vi "DSP模拟量输入.vi"() -> ()   [LabVIEW 2010]
panel:
  out "DSP_R_16_5":sgl format="%.2f"
  out "DSP_R_16_4":sgl format="%.2f"
  out "DSP_R_16_3":sgl format="%.2f"
  out "DSP_R_16_2":sgl format="%.2f"
  out "DSP_R_16_1":sgl format="%.2f"
  out "DSP_R_15_5":sgl format="%.2f"
  out "DSP_R_15_4":sgl format="%.2f"
  out "DSP_R_15_3":sgl format="%.2f"
  out "DSP_R_15_2":sgl format="%.2f"
  out "DSP_R_15_1":sgl format="%.2f"
  out "DSP_R_14_5":sgl format="%.2f"
  out "DSP_R_14_4":sgl format="%.2f"
  out "DSP_R_14_3":sgl format="%.2f"
  out "DSP_R_14_2":sgl format="%.2f"
  out "DSP_R_14_1":sgl format="%.2f"
  out "DSP_R_13_5":sgl format="%.2f"
  out "DSP_R_13_4":sgl format="%.2f"
  out "DSP_R_13_3":sgl format="%.2f"
  out "DSP_R_13_2":sgl format="%.2f"
  out "DSP_R_13_1":sgl format="%.2f"
  out "DSP_R_12_5":sgl format="%.2f"
  out "DSP_R_12_4":sgl format="%.2f"
  out "DSP_R_12_3":sgl format="%.2f"
  out "DSP_R_12_2":sgl format="%.2f"
  out "DSP_R_12_1":sgl format="%.2f"
  out "DSP_R_11_5":sgl format="%.2f"
  out "DSP_R_11_4":sgl format="%.2f"
  out "DSP_R_11_3":sgl format="%.2f"
  out "DSP_R_11_2":sgl format="%.2f"
  out "DSP_R_11_1":sgl format="%.2f"
  out "DSP_R_10_5":sgl format="%.2f"
  out "DSP_R_10_4":sgl format="%.2f"
  out "DSP_R_10_3":sgl format="%.2f"
  out "DSP_R_10_2":sgl format="%.2f"
  out "DSP_R_10_1":sgl format="%.2f"
  out "DSP_R_9_5":sgl format="%.2f"
  out "DSP_R_9_4":sgl format="%.2f"
  out "DSP_R_9_3":sgl format="%.2f"
  out "DSP_R_9_2":sgl format="%.2f"
  out "DSP_R_9_1":sgl format="%.2f"
  out "DSP_R_8_5":sgl format="%.2f"
  out "DSP_R_8_4":sgl format="%.2f"
  out "DSP_R_8_3":sgl format="%.2f"
  out "DSP_R_8_2":sgl format="%.2f"
  out "DSP_R_8_1":sgl format="%.2f"
  out "DSP_R_7_5":sgl format="%.2f"
  out "DSP_R_7_4":sgl format="%.2f"
  out "DSP_R_7_3":sgl format="%.2f"
  out "DSP_R_7_2":sgl format="%.2f"
  out "DSP_R_7_1":sgl format="%.2f"
  out "DSP_R_6_5":sgl format="%.2f"
  out "DSP_R_6_4":sgl format="%.2f"
  out "DSP_R_6_3":sgl format="%.2f"
  out "DSP_R_6_2":sgl format="%.2f"
  out "DSP_R_6_1":sgl format="%.2f"
  out "DSP_R_5_5":sgl format="%.2f"
  out "DSP_R_5_4":sgl format="%.2f"
  out "DSP_R_5_3":sgl format="%.2f"
  out "DSP_R_5_2":sgl format="%.2f"
  out "DSP_R_5_1":sgl format="%.2f"
  out "DSP_R_4_5":sgl format="%.2f"
  out "DSP_R_4_4":sgl format="%.2f"
  out "DSP_R_4_3":sgl format="%.2f"
  out "DSP_R_4_2":sgl format="%.2f"
  out "DSP_R_4_1":sgl format="%.2f"
  out "DSP_R_3_5":sgl format="%.2f"
  out "DSP_R_3_4":sgl format="%.2f"
  out "DSP_R_3_3":sgl format="%.2f"
  out "DSP_R_3_2":sgl format="%.2f"
  out "DSP_R_3_1":sgl format="%.2f"
  out "DSP_R_2_5":sgl format="%.2f"
  out "DSP_R_2_4":sgl format="%.2f"
  out "DSP_R_2_3":sgl format="%.2f"
  out "DSP_R_2_2":sgl format="%.2f"
  out "DSP_R_2_1":sgl format="%.2f"
  out "DSP_R_1_5":sgl format="%.2f"
  out "DSP_R_1_4":sgl format="%.2f"
  out "DSP_R_1_3":sgl format="%.2f"
  out "DSP_R_1_2":sgl format="%.2f"
  out "DSP_R_1_1":sgl format="%.2f"
  out "合格？":bool[][](array[boolean])
  out "开始时间":dbl format="%#.0f"
  out "测试结论":string
  out "light_16":bool
  out "light_15":bool
  out "light_14":bool
  out "light_13":bool
  out "light_12":bool
  out "light_11":bool
  out "light_10":bool
  out "light_9":bool
  out "light_8":bool
  out "light_7":bool
  out "light_6":bool
  out "light_5":bool
  out "light_4":bool
  out "light_3":bool
  out "light_2":bool
  out "light_1":bool
  out "退出？":bool
  in  "btn_反选":bool
  in  "btn_全选":bool
  in  "DSP_16_5":sgl format="%.2f"
  in  "DSP_16_4":sgl format="%.2f"
  in  "DSP_16_3":sgl format="%.2f"
  in  "DSP_16_2":sgl format="%.2f"
  in  "DSP_16_1":sgl format="%.2f"
  in  "DSP_15_5":sgl format="%.2f"
  in  "DSP_15_4":sgl format="%.2f"
  in  "DSP_15_3":sgl format="%.2f"
  in  "DSP_15_2":sgl format="%.2f"
  in  "单选_DSP_16":bool
  in  "单选_DSP_15":bool
  in  "DSP_15_1":sgl format="%.2f"
  in  "DSP_14_5":sgl format="%.2f"
  in  "DSP_14_4":sgl format="%.2f"
  in  "DSP_14_3":sgl format="%.2f"
  in  "DSP_14_2":sgl format="%.2f"
  in  "DSP_6_14":sgl format="%.2f"
  in  "DSP_13_5":sgl format="%.2f"
  in  "DSP_13_4":sgl format="%.2f"
  in  "DSP_13_3":sgl format="%.2f"
  in  "DSP_13_2":sgl format="%.2f"
  in  "单选_DSP_14":bool
  in  "单选_DSP_13":bool
  in  "DSP_13_1":sgl format="%.2f"
  in  "DSP_12_5":sgl format="%.2f"
  in  "DSP_12_4":sgl format="%.2f"
  in  "DSP_12_3":sgl format="%.2f"
  in  "DSP_12_2":sgl format="%.2f"
  in  "DSP_12_1":sgl format="%.2f"
  in  "DSP_11_5":sgl format="%.2f"
  in  "DSP_11_4":sgl format="%.2f"
  in  "DSP_11_3":sgl format="%.2f"
  in  "DSP_11_2":sgl format="%.2f"
  in  "单选_DSP_12":bool
  in  "单选_DSP_11":bool
  in  "DSP_11_1":sgl format="%.2f"
  in  "DSP_10_5":sgl format="%.2f"
  in  "DSP_10_4":sgl format="%.2f"
  in  "DSP_10_3":sgl format="%.2f"
  in  "DSP_10_2":sgl format="%.2f"
  in  "DSP_10_1":sgl format="%.2f"
  in  "DSP_9_5":sgl format="%.2f"
  in  "DSP_9_4":sgl format="%.2f"
  in  "DSP_9_3":sgl format="%.2f"
  in  "DSP_9_2":sgl format="%.2f"
  in  "单选_DSP_10":bool
  in  "单选_DSP_9":bool
  in  "DSP_9_1":sgl format="%.2f"
  in  "DSP_8_5":sgl format="%.2f"
  in  "DSP_8_4":sgl format="%.2f"
  in  "DSP_8_3":sgl format="%.2f"
  in  "DSP_8_2":sgl format="%.2f"
  in  "DSP_8_1":sgl format="%.2f"
  in  "DSP_7_5":sgl format="%.2f"
  in  "DSP_7_4":sgl format="%.2f"
  in  "DSP_7_3":sgl format="%.2f"
  in  "DSP_7_2":sgl format="%.2f"
  in  "单选_DSP_8":bool
  in  "单选_DSP_7":bool
  in  "DSP_7_1":sgl format="%.2f"
  in  "DSP_6_5":sgl format="%.2f"
  in  "DSP_6_4":sgl format="%.2f"
  in  "DSP_6_3":sgl format="%.2f"
  in  "DSP_6_2":sgl format="%.2f"
  in  "DSP_6_1":sgl format="%.2f"
  in  "DSP_5_5":sgl format="%.2f"
  in  "DSP_5_4":sgl format="%.2f"
  in  "DSP_5_3":sgl format="%.2f"
  in  "DSP_5_2":sgl format="%.2f"
  in  "单选_DSP_6":bool
  in  "单选_DSP_5":bool
  in  "DSP_5_1":sgl format="%.2f"
  in  "DSP_4_5":sgl format="%.2f"
  in  "DSP_4_4":sgl format="%.2f"
  in  "DSP_4_3":sgl format="%.2f"
  in  "DSP_4_2":sgl format="%.2f"
  in  "DSP_4_1":sgl format="%.2f"
  in  "DSP_3_5":sgl format="%.2f"
  in  "DSP_3_4":sgl format="%.2f"
  in  "DSP_3_3":sgl format="%.2f"
  in  "DSP_3_2":sgl format="%.2f"
  in  "单选_DSP_4":bool
  in  "单选_DSP_3":bool
  in  "DSP_3_1":sgl format="%.2f"
  in  "DSP_2_5":sgl format="%.2f"
  in  "DSP_2_4":sgl format="%.2f"
  in  "DSP_2_3":sgl format="%.2f"
  in  "DSP_2_2":sgl format="%.2f"
  in  "DSP_2_1":sgl format="%.2f"
  in  "DSP_1_5":sgl format="%.2f"
  in  "DSP_1_4":sgl format="%.2f"
  in  "DSP_1_3":sgl format="%.2f"
  in  "DSP_1_2":sgl format="%.2f"
  in  "单选_DSP_2":bool
  in  "单选_DSP_1":bool
  in  "DSP_1_1":sgl format="%.2f"
  in  "btn_取消":bool
  in  "btn_开始测试":bool
  # "第1路"
  # "输入值："
  # "输入值："
  # "第2路"
  # "第3路"
  # "输入值："
  # "输入值："
  # "第4路"
  # "第5路"
  # "输入值："
  # "输入值："
  # "第6路"
  # "第7路"
  # "输入值："
  # "输入值："
  # "第8路"
  # "第9路"
  # "输入值："
  # "输入值："
  # "第10路"
  # "第11路"
  # "输入值："
  # "输入值："
  # "第12路"
  # "第13路"
  # "输入值："
  # "输入值："
  # "第14路"
  # "第15路"
  # "输入值："
  # "输入值："
  # "第16路"
  # "测试结论："
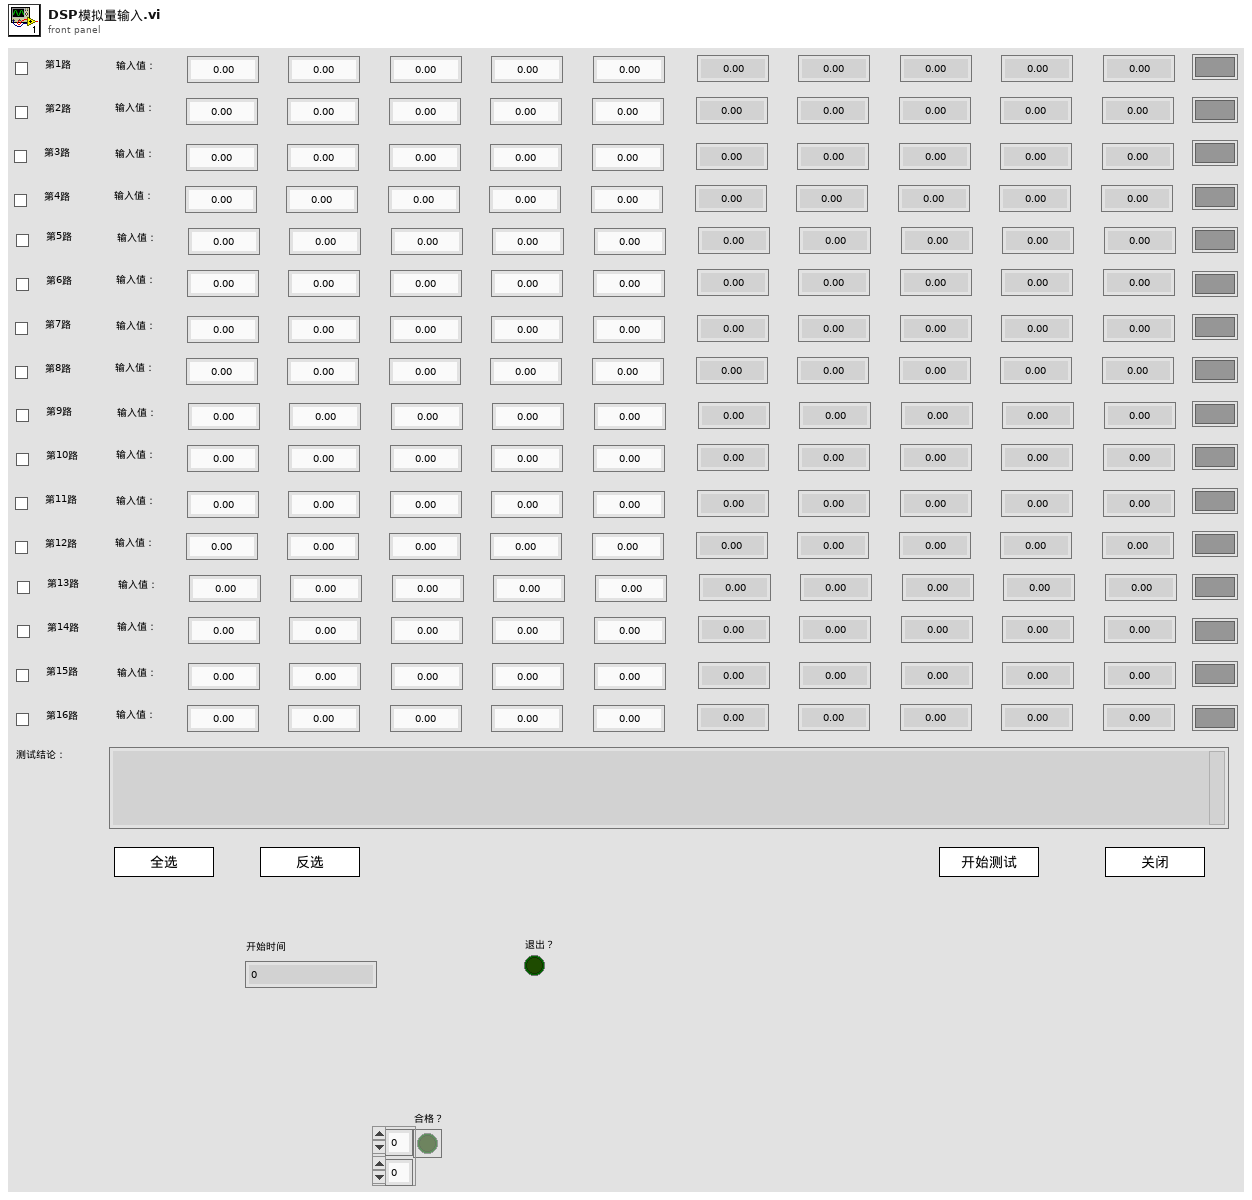
[diagram p1: front panel]
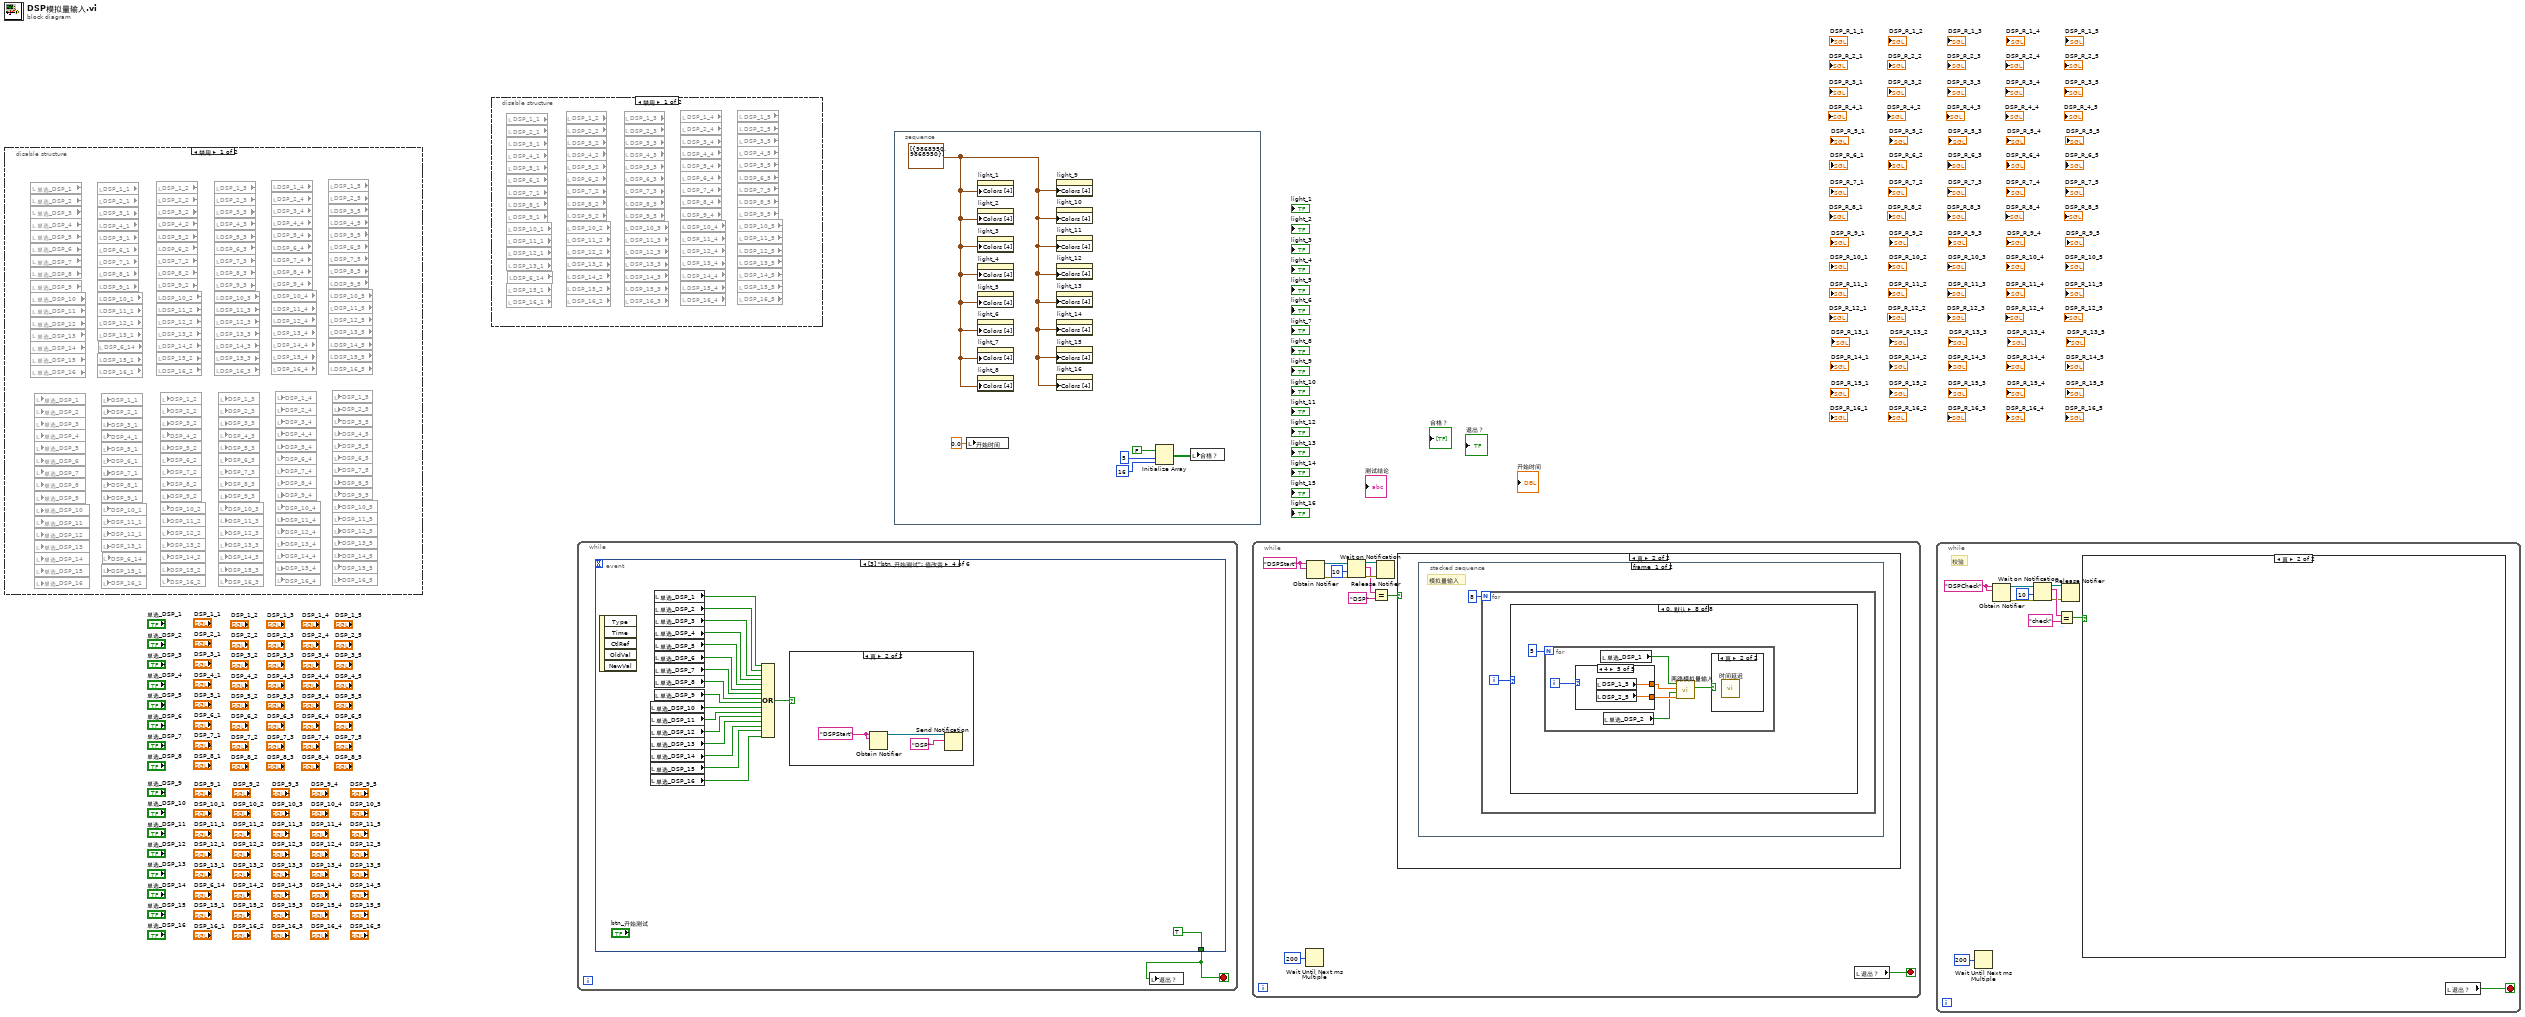
[diagram p0: block diagram]
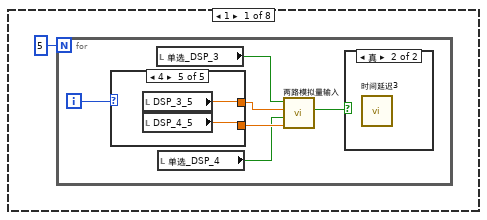
[diagram p5: hidden frame]
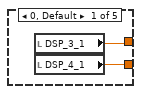
[diagram p7: hidden frame]
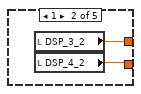
[diagram p8: hidden frame]
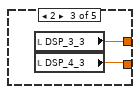
[diagram p9: hidden frame]
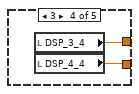
[diagram p10: hidden frame]
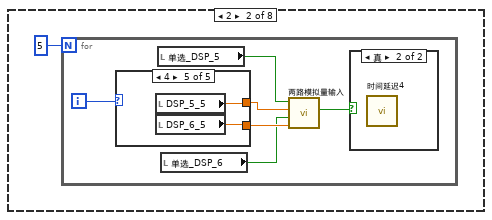
[diagram p11: hidden frame]
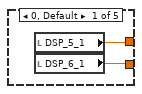
[diagram p13: hidden frame]
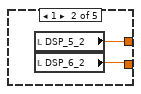
[diagram p14: hidden frame]
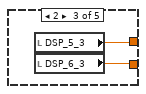
[diagram p15: hidden frame]
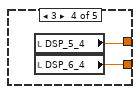
[diagram p16: hidden frame]
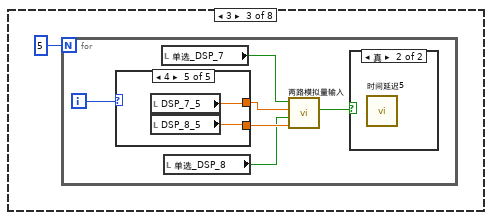
[diagram p17: hidden frame]
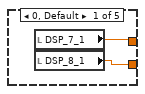
[diagram p19: hidden frame]
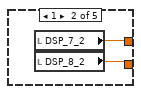
[diagram p20: hidden frame]
diagram:
  n1 = disable-structure shown="禁用" {
    frame Disabled {
      n2 = local read "单选_DSP_1"() -> ()  [unwired: 1 out]
      n3 = local read "单选_DSP_2"() -> ()  [unwired: 1 out]
      n4 = local read "单选_DSP_3"() -> ()  [unwired: 1 out]
      n5 = local read "单选_DSP_4"() -> ()  [unwired: 1 out]
      n6 = local read "单选_DSP_5"() -> ()  [unwired: 1 out]
      n7 = local read "单选_DSP_6"() -> ()  [unwired: 1 out]
      n8 = local read "单选_DSP_7"() -> ()  [unwired: 1 out]
      n9 = local read "单选_DSP_8"() -> ()  [unwired: 1 out]
      n10 = local read "单选_DSP_9"() -> ()  [unwired: 1 out]
      n11 = local read "单选_DSP_10"() -> ()  [unwired: 1 out]
      n12 = local read "单选_DSP_11"() -> ()  [unwired: 1 out]
      n13 = local read "单选_DSP_12"() -> ()  [unwired: 1 out]
      n14 = local read "单选_DSP_13"() -> ()  [unwired: 1 out]
      n15 = local read "单选_DSP_14"() -> ()  [unwired: 1 out]
      n16 = local read "单选_DSP_15"() -> ()  [unwired: 1 out]
      n17 = local read "单选_DSP_16"() -> ()  [unwired: 1 out]
      n18 = local read "单选_DSP_1"() -> ()  [unwired: 1 in]
      n19 = local read "单选_DSP_2"() -> ()  [unwired: 1 in]
      n20 = local read "单选_DSP_3"() -> ()  [unwired: 1 in]
      n21 = local read "单选_DSP_4"() -> ()  [unwired: 1 in]
      n22 = local read "单选_DSP_5"() -> ()  [unwired: 1 in]
      n23 = local read "单选_DSP_6"() -> ()  [unwired: 1 in]
      n24 = local read "单选_DSP_7"() -> ()  [unwired: 1 in]
      n25 = local read "单选_DSP_8"() -> ()  [unwired: 1 in]
      n26 = local read "单选_DSP_9"() -> ()  [unwired: 1 in]
      n27 = local read "单选_DSP_10"() -> ()  [unwired: 1 in]
      n28 = local read "单选_DSP_11"() -> ()  [unwired: 1 in]
      n29 = local read "单选_DSP_12"() -> ()  [unwired: 1 in]
      n30 = local read "单选_DSP_13"() -> ()  [unwired: 1 in]
      n31 = local read "单选_DSP_14"() -> ()  [unwired: 1 in]
      n32 = local read "单选_DSP_15"() -> ()  [unwired: 1 in]
      n33 = local read "单选_DSP_16"() -> ()  [unwired: 1 in]
      n34 = local read "DSP_1_1"() -> ()  [unwired: 1 out]
      n35 = local read "DSP_2_1"() -> ()  [unwired: 1 out]
      n36 = local read "DSP_3_1"() -> ()  [unwired: 1 out]
      n37 = local read "DSP_4_1"() -> ()  [unwired: 1 out]
      n38 = local read "DSP_5_1"() -> ()  [unwired: 1 out]
      n39 = local read "DSP_6_1"() -> ()  [unwired: 1 out]
      n40 = local read "DSP_7_1"() -> ()  [unwired: 1 out]
      n41 = local read "DSP_8_1"() -> ()  [unwired: 1 out]
      n42 = local read "DSP_9_1"() -> ()  [unwired: 1 out]
      n43 = local read "DSP_10_1"() -> ()  [unwired: 1 out]
      n44 = local read "DSP_11_1"() -> ()  [unwired: 1 out]
      n45 = local read "DSP_12_1"() -> ()  [unwired: 1 out]
      n46 = local read "DSP_13_1"() -> ()  [unwired: 1 out]
      n47 = local read "DSP_15_1"() -> ()  [unwired: 1 out]
      n48 = local read "DSP_16_1"() -> ()  [unwired: 1 out]
      n49 = local read "DSP_6_14"() -> ()  [unwired: 1 out]
      n50 = local read "DSP_1_1"() -> ()  [unwired: 1 in]
      n51 = local read "DSP_2_1"() -> ()  [unwired: 1 in]
      n52 = local read "DSP_3_1"() -> ()  [unwired: 1 in]
      n53 = local read "DSP_4_1"() -> ()  [unwired: 1 in]
      n54 = local read "DSP_5_1"() -> ()  [unwired: 1 in]
      n55 = local read "DSP_6_1"() -> ()  [unwired: 1 in]
      n56 = local read "DSP_7_1"() -> ()  [unwired: 1 in]
      n57 = local read "DSP_8_1"() -> ()  [unwired: 1 in]
      n58 = local read "DSP_9_1"() -> ()  [unwired: 1 in]
      n59 = local read "DSP_10_1"() -> ()  [unwired: 1 in]
      n60 = local read "DSP_11_1"() -> ()  [unwired: 1 in]
      n61 = local read "DSP_12_1"() -> ()  [unwired: 1 in]
      n62 = local read "DSP_13_1"() -> ()  [unwired: 1 in]
      n63 = local read "DSP_15_1"() -> ()  [unwired: 1 in]
      n64 = local read "DSP_16_1"() -> ()  [unwired: 1 in]
      n65 = local read "DSP_6_14"() -> ()  [unwired: 1 in]
      n66 = local read "DSP_1_2"() -> ()  [unwired: 1 out]
      n67 = local read "DSP_2_2"() -> ()  [unwired: 1 out]
      n68 = local read "DSP_3_2"() -> ()  [unwired: 1 out]
      n69 = local read "DSP_4_2"() -> ()  [unwired: 1 out]
      n70 = local read "DSP_5_2"() -> ()  [unwired: 1 out]
      n71 = local read "DSP_6_2"() -> ()  [unwired: 1 out]
      n72 = local read "DSP_7_2"() -> ()  [unwired: 1 out]
      n73 = local read "DSP_8_2"() -> ()  [unwired: 1 out]
      n74 = local read "DSP_9_2"() -> ()  [unwired: 1 out]
      n75 = local read "DSP_10_2"() -> ()  [unwired: 1 out]
      n76 = local read "DSP_11_2"() -> ()  [unwired: 1 out]
      n77 = local read "DSP_12_2"() -> ()  [unwired: 1 out]
      n78 = local read "DSP_13_2"() -> ()  [unwired: 1 out]
      n79 = local read "DSP_14_2"() -> ()  [unwired: 1 out]
      n80 = local read "DSP_15_2"() -> ()  [unwired: 1 out]
      n81 = local read "DSP_16_2"() -> ()  [unwired: 1 out]
      n82 = local read "DSP_1_2"() -> ()  [unwired: 1 in]
      n83 = local read "DSP_2_2"() -> ()  [unwired: 1 in]
      n84 = local read "DSP_3_2"() -> ()  [unwired: 1 in]
      n85 = local read "DSP_4_2"() -> ()  [unwired: 1 in]
      n86 = local read "DSP_5_2"() -> ()  [unwired: 1 in]
      n87 = local read "DSP_6_2"() -> ()  [unwired: 1 in]
      n88 = local read "DSP_7_2"() -> ()  [unwired: 1 in]
      n89 = local read "DSP_8_2"() -> ()  [unwired: 1 in]
      n90 = local read "DSP_9_2"() -> ()  [unwired: 1 in]
      n91 = local read "DSP_10_2"() -> ()  [unwired: 1 in]
      n92 = local read "DSP_11_2"() -> ()  [unwired: 1 in]
      n93 = local read "DSP_12_2"() -> ()  [unwired: 1 in]
      n94 = local read "DSP_13_2"() -> ()  [unwired: 1 in]
      n95 = local read "DSP_14_2"() -> ()  [unwired: 1 in]
      n96 = local read "DSP_15_2"() -> ()  [unwired: 1 in]
      n97 = local read "DSP_16_2"() -> ()  [unwired: 1 in]
      n98 = local read "DSP_1_3"() -> ()  [unwired: 1 out]
      n99 = local read "DSP_2_3"() -> ()  [unwired: 1 out]
      n100 = local read "DSP_3_3"() -> ()  [unwired: 1 out]
      n101 = local read "DSP_4_3"() -> ()  [unwired: 1 out]
      n102 = local read "DSP_5_3"() -> ()  [unwired: 1 out]
      n103 = local read "DSP_6_3"() -> ()  [unwired: 1 out]
      n104 = local read "DSP_7_3"() -> ()  [unwired: 1 out]
      n105 = local read "DSP_8_3"() -> ()  [unwired: 1 out]
      n106 = local read "DSP_9_3"() -> ()  [unwired: 1 out]
      n107 = local read "DSP_10_3"() -> ()  [unwired: 1 out]
      n108 = local read "DSP_11_3"() -> ()  [unwired: 1 out]
      n109 = local read "DSP_12_3"() -> ()  [unwired: 1 out]
      n110 = local read "DSP_13_3"() -> ()  [unwired: 1 out]
      n111 = local read "DSP_14_3"() -> ()  [unwired: 1 out]
      n112 = local read "DSP_15_3"() -> ()  [unwired: 1 out]
      n113 = local read "DSP_16_3"() -> ()  [unwired: 1 out]
      n114 = local read "DSP_1_3"() -> ()  [unwired: 1 in]
      n115 = local read "DSP_2_3"() -> ()  [unwired: 1 in]
      n116 = local read "DSP_3_3"() -> ()  [unwired: 1 in]
      n117 = local read "DSP_4_3"() -> ()  [unwired: 1 in]
      n118 = local read "DSP_5_3"() -> ()  [unwired: 1 in]
      n119 = local read "DSP_6_3"() -> ()  [unwired: 1 in]
      n120 = local read "DSP_7_3"() -> ()  [unwired: 1 in]
      n121 = local read "DSP_8_3"() -> ()  [unwired: 1 in]
      n122 = local read "DSP_9_3"() -> ()  [unwired: 1 in]
      n123 = local read "DSP_10_3"() -> ()  [unwired: 1 in]
      n124 = local read "DSP_11_3"() -> ()  [unwired: 1 in]
      n125 = local read "DSP_12_3"() -> ()  [unwired: 1 in]
      n126 = local read "DSP_13_3"() -> ()  [unwired: 1 in]
      n127 = local read "DSP_14_3"() -> ()  [unwired: 1 in]
      n128 = local read "DSP_15_3"() -> ()  [unwired: 1 in]
      n129 = local read "DSP_16_3"() -> ()  [unwired: 1 in]
      n130 = local read "DSP_1_4"() -> ()  [unwired: 1 out]
      n131 = local read "DSP_2_4"() -> ()  [unwired: 1 out]
      n132 = local read "DSP_3_4"() -> ()  [unwired: 1 out]
      n133 = local read "DSP_4_4"() -> ()  [unwired: 1 out]
      n134 = local read "DSP_5_4"() -> ()  [unwired: 1 out]
      n135 = local read "DSP_6_4"() -> ()  [unwired: 1 out]
      n136 = local read "DSP_7_4"() -> ()  [unwired: 1 out]
      n137 = local read "DSP_8_4"() -> ()  [unwired: 1 out]
      n138 = local read "DSP_9_4"() -> ()  [unwired: 1 out]
      n139 = local read "DSP_10_4"() -> ()  [unwired: 1 out]
      n140 = local read "DSP_11_4"() -> ()  [unwired: 1 out]
      n141 = local read "DSP_12_4"() -> ()  [unwired: 1 out]
      n142 = local read "DSP_13_4"() -> ()  [unwired: 1 out]
      n143 = local read "DSP_14_4"() -> ()  [unwired: 1 out]
      n144 = local read "DSP_15_4"() -> ()  [unwired: 1 out]
      n145 = local read "DSP_16_4"() -> ()  [unwired: 1 out]
      n146 = local read "DSP_1_4"() -> ()  [unwired: 1 in]
      n147 = local read "DSP_2_4"() -> ()  [unwired: 1 in]
      n148 = local read "DSP_3_4"() -> ()  [unwired: 1 in]
      n149 = local read "DSP_4_4"() -> ()  [unwired: 1 in]
      n150 = local read "DSP_5_4"() -> ()  [unwired: 1 in]
      n151 = local read "DSP_6_4"() -> ()  [unwired: 1 in]
      n152 = local read "DSP_7_4"() -> ()  [unwired: 1 in]
      n153 = local read "DSP_8_4"() -> ()  [unwired: 1 in]
      n154 = local read "DSP_9_4"() -> ()  [unwired: 1 in]
      n155 = local read "DSP_10_4"() -> ()  [unwired: 1 in]
      n156 = local read "DSP_11_4"() -> ()  [unwired: 1 in]
      n157 = local read "DSP_12_4"() -> ()  [unwired: 1 in]
      n158 = local read "DSP_13_4"() -> ()  [unwired: 1 in]
      n159 = local read "DSP_14_4"() -> ()  [unwired: 1 in]
      n160 = local read "DSP_15_4"() -> ()  [unwired: 1 in]
      n161 = local read "DSP_16_4"() -> ()  [unwired: 1 in]
      n162 = local read "DSP_1_5"() -> ()  [unwired: 1 out]
      n163 = local read "DSP_2_5"() -> ()  [unwired: 1 out]
      n164 = local read "DSP_3_5"() -> ()  [unwired: 1 out]
      n165 = local read "DSP_4_5"() -> ()  [unwired: 1 out]
      n166 = local read "DSP_5_5"() -> ()  [unwired: 1 out]
      n167 = local read "DSP_6_5"() -> ()  [unwired: 1 out]
      n168 = local read "DSP_7_5"() -> ()  [unwired: 1 out]
      n169 = local read "DSP_8_5"() -> ()  [unwired: 1 out]
      n170 = local read "DSP_9_5"() -> ()  [unwired: 1 out]
      n171 = local read "DSP_10_5"() -> ()  [unwired: 1 out]
      n172 = local read "DSP_11_5"() -> ()  [unwired: 1 out]
      n173 = local read "DSP_12_5"() -> ()  [unwired: 1 out]
      n174 = local read "DSP_13_5"() -> ()  [unwired: 1 out]
      n175 = local read "DSP_14_5"() -> ()  [unwired: 1 out]
      n176 = local read "DSP_15_5"() -> ()  [unwired: 1 out]
      n177 = local read "DSP_16_5"() -> ()  [unwired: 1 out]
      n178 = local read "DSP_1_5"() -> ()  [unwired: 1 in]
      n179 = local read "DSP_2_5"() -> ()  [unwired: 1 in]
      n180 = local read "DSP_3_5"() -> ()  [unwired: 1 in]
      n181 = local read "DSP_4_5"() -> ()  [unwired: 1 in]
      n182 = local read "DSP_5_5"() -> ()  [unwired: 1 in]
      n183 = local read "DSP_6_5"() -> ()  [unwired: 1 in]
      n184 = local read "DSP_7_5"() -> ()  [unwired: 1 in]
      n185 = local read "DSP_8_5"() -> ()  [unwired: 1 in]
      n186 = local read "DSP_9_5"() -> ()  [unwired: 1 in]
      n187 = local read "DSP_10_5"() -> ()  [unwired: 1 in]
      n188 = local read "DSP_11_5"() -> ()  [unwired: 1 in]
      n189 = local read "DSP_12_5"() -> ()  [unwired: 1 in]
      n190 = local read "DSP_13_5"() -> ()  [unwired: 1 in]
      n191 = local read "DSP_14_5"() -> ()  [unwired: 1 in]
      n192 = local read "DSP_15_5"() -> ()  [unwired: 1 in]
      n193 = local read "DSP_16_5"() -> ()  [unwired: 1 in]
    }
    frame Enabled {
    }
  }
  n194 = disable-structure shown="禁用" {
    frame Disabled {
      n195 = local read "DSP_1_1"() -> ()  [unwired: 1 out]
      n196 = local read "DSP_2_1"() -> ()  [unwired: 1 out]
      n197 = local read "DSP_3_1"() -> ()  [unwired: 1 out]
      n198 = local read "DSP_4_1"() -> ()  [unwired: 1 out]
      n199 = local read "DSP_5_1"() -> ()  [unwired: 1 out]
      n200 = local read "DSP_6_1"() -> ()  [unwired: 1 out]
      n201 = local read "DSP_7_1"() -> ()  [unwired: 1 out]
      n202 = local read "DSP_8_1"() -> ()  [unwired: 1 out]
      n203 = local read "DSP_9_1"() -> ()  [unwired: 1 out]
      n204 = local read "DSP_10_1"() -> ()  [unwired: 1 out]
      n205 = local read "DSP_11_1"() -> ()  [unwired: 1 out]
      n206 = local read "DSP_12_1"() -> ()  [unwired: 1 out]
      n207 = local read "DSP_13_1"() -> ()  [unwired: 1 out]
      n208 = local read "DSP_15_1"() -> ()  [unwired: 1 out]
      n209 = local read "DSP_16_1"() -> ()  [unwired: 1 out]
      n210 = local read "DSP_6_14"() -> ()  [unwired: 1 out]
      n211 = local read "DSP_1_2"() -> ()  [unwired: 1 out]
      n212 = local read "DSP_2_2"() -> ()  [unwired: 1 out]
      n213 = local read "DSP_3_2"() -> ()  [unwired: 1 out]
      n214 = local read "DSP_4_2"() -> ()  [unwired: 1 out]
      n215 = local read "DSP_5_2"() -> ()  [unwired: 1 out]
      n216 = local read "DSP_6_2"() -> ()  [unwired: 1 out]
      n217 = local read "DSP_7_2"() -> ()  [unwired: 1 out]
      n218 = local read "DSP_8_2"() -> ()  [unwired: 1 out]
      n219 = local read "DSP_9_2"() -> ()  [unwired: 1 out]
      n220 = local read "DSP_10_2"() -> ()  [unwired: 1 out]
      n221 = local read "DSP_11_2"() -> ()  [unwired: 1 out]
      n222 = local read "DSP_12_2"() -> ()  [unwired: 1 out]
      n223 = local read "DSP_13_2"() -> ()  [unwired: 1 out]
      n224 = local read "DSP_14_2"() -> ()  [unwired: 1 out]
      n225 = local read "DSP_15_2"() -> ()  [unwired: 1 out]
      n226 = local read "DSP_16_2"() -> ()  [unwired: 1 out]
      n227 = local read "DSP_1_3"() -> ()  [unwired: 1 out]
      n228 = local read "DSP_2_3"() -> ()  [unwired: 1 out]
      n229 = local read "DSP_3_3"() -> ()  [unwired: 1 out]
      n230 = local read "DSP_4_3"() -> ()  [unwired: 1 out]
      n231 = local read "DSP_5_3"() -> ()  [unwired: 1 out]
      n232 = local read "DSP_6_3"() -> ()  [unwired: 1 out]
      n233 = local read "DSP_7_3"() -> ()  [unwired: 1 out]
      n234 = local read "DSP_8_3"() -> ()  [unwired: 1 out]
      n235 = local read "DSP_9_3"() -> ()  [unwired: 1 out]
      n236 = local read "DSP_10_3"() -> ()  [unwired: 1 out]
      n237 = local read "DSP_11_3"() -> ()  [unwired: 1 out]
      n238 = local read "DSP_12_3"() -> ()  [unwired: 1 out]
      n239 = local read "DSP_13_3"() -> ()  [unwired: 1 out]
      n240 = local read "DSP_14_3"() -> ()  [unwired: 1 out]
      n241 = local read "DSP_15_3"() -> ()  [unwired: 1 out]
      n242 = local read "DSP_16_3"() -> ()  [unwired: 1 out]
      n243 = local read "DSP_1_4"() -> ()  [unwired: 1 out]
      n244 = local read "DSP_2_4"() -> ()  [unwired: 1 out]
      n245 = local read "DSP_3_4"() -> ()  [unwired: 1 out]
      n246 = local read "DSP_4_4"() -> ()  [unwired: 1 out]
      n247 = local read "DSP_5_4"() -> ()  [unwired: 1 out]
      n248 = local read "DSP_6_4"() -> ()  [unwired: 1 out]
      n249 = local read "DSP_7_4"() -> ()  [unwired: 1 out]
      n250 = local read "DSP_8_4"() -> ()  [unwired: 1 out]
      n251 = local read "DSP_9_4"() -> ()  [unwired: 1 out]
      n252 = local read "DSP_10_4"() -> ()  [unwired: 1 out]
      n253 = local read "DSP_11_4"() -> ()  [unwired: 1 out]
      n254 = local read "DSP_12_4"() -> ()  [unwired: 1 out]
      n255 = local read "DSP_13_4"() -> ()  [unwired: 1 out]
      n256 = local read "DSP_14_4"() -> ()  [unwired: 1 out]
      n257 = local read "DSP_15_4"() -> ()  [unwired: 1 out]
      n258 = local read "DSP_16_4"() -> ()  [unwired: 1 out]
      n259 = local read "DSP_1_5"() -> ()  [unwired: 1 out]
      n260 = local read "DSP_2_5"() -> ()  [unwired: 1 out]
      n261 = local read "DSP_3_5"() -> ()  [unwired: 1 out]
      n262 = local read "DSP_4_5"() -> ()  [unwired: 1 out]
      n263 = local read "DSP_5_5"() -> ()  [unwired: 1 out]
      n264 = local read "DSP_6_5"() -> ()  [unwired: 1 out]
      n265 = local read "DSP_7_5"() -> ()  [unwired: 1 out]
      n266 = local read "DSP_8_5"() -> ()  [unwired: 1 out]
      n267 = local read "DSP_9_5"() -> ()  [unwired: 1 out]
      n268 = local read "DSP_10_5"() -> ()  [unwired: 1 out]
      n269 = local read "DSP_11_5"() -> ()  [unwired: 1 out]
      n270 = local read "DSP_12_5"() -> ()  [unwired: 1 out]
      n271 = local read "DSP_13_5"() -> ()  [unwired: 1 out]
      n272 = local read "DSP_14_5"() -> ()  [unwired: 1 out]
      n273 = local read "DSP_15_5"() -> ()  [unwired: 1 out]
      n274 = local read "DSP_16_5"() -> ()  [unwired: 1 out]
    }
    frame Enabled {
    }
  }
  n275 = while {
    stop <- w1 stop-if-true
    n276 = event shown="[3] \"btn_开始测试\": 值改变" {
      selector: _ -> [_ _ _ _ _ _]
      dyn-events: _ -> [_ _ _ _ _ _]
      timeout: _ -> [_ _ _ _ _ _]
      tunnel: [_ TRUE TRUE TRUE _ _] -> w1
      event Timeout {
        n277 = event-data() -> ()  [unwired: 1 in, 2 out]
      }
      event Panel Close {
        n278 = event-data() -> ()  [unwired: 1 in, 3 out]
      }
      event "btn_取消": Value Change {
        n279 = event-data() -> ()  [unwired: 1 in, 5 out]
      }
      event "btn_开始测试": Value Change {
        n280 = event-data() -> ()  [unwired: 1 in, 5 out]
        n281 = local read "单选_DSP_10"() -> (w11:bool)
        n282 = local read "单选_DSP_11"() -> (w10:bool)
        n283 = local read "单选_DSP_12"() -> (w9:bool)
        n284 = local read "单选_DSP_13"() -> (w8:bool)
        n285 = local read "单选_DSP_14"() -> (w7:bool)
        n286 = local read "单选_DSP_15"() -> (w6:bool)
        n287 = local read "单选_DSP_16"() -> (w5:bool)
        n288 = local read "单选_DSP_1"() -> (w20:bool)
        n289 = local read "单选_DSP_2"() -> (w19:bool)
        n290 = local read "单选_DSP_3"() -> (w18:bool)
        n291 = local read "单选_DSP_4"() -> (w17:bool)
        n292 = local read "单选_DSP_5"() -> (w16:bool)
        n293 = local read "单选_DSP_6"() -> (w15:bool)
        n294 = local read "单选_DSP_7"() -> (w14:bool)
        n295 = local read "单选_DSP_8"() -> (w13:bool)
        n296 = local read "单选_DSP_9"() -> (w12:bool)
        n297 = Compound Arithmetic op=OR(w20, w19, w18, w17, w16, w15, w14, w13, w12, w11, w10, w9, w8, w7, w6, w5) -> (w4:bool)
        n298 = case shown="真" w4 {
          frame False {
            n299 = call "显示对话框信息"() -> ()  [unwired: 10 in, 2 out]
          }
          frame True {
            w23 = "DSPStart" ("名称（未命名）")
            n300 = Obtain Notifier(name (unnamed)=w23, notification data type=w23) -> (notifier out=w22:refnum<notifier>)  [unwired: 2 in, 2 out]
            n301 = Send Notification(notification="DSP" ("通知"), notifier=w22) -> ()  [unwired: 1 in, 2 out]
          }
        }
      }
      event "btn_全选": Value Change {
        w25 = TRUE ("单选_AD_1")
        n302 = event-data() -> ()  [unwired: 1 in, 5 out]
        n303 = local write "单选_DSP_1"(w25) -> ()
        n304 = local write "单选_DSP_2"(w25) -> ()
        n305 = local write "单选_DSP_3"(w25) -> ()
        n306 = local write "单选_DSP_4"(w25) -> ()
        n307 = local write "单选_DSP_5"(w25) -> ()
        n308 = local write "单选_DSP_6"(w25) -> ()
        n309 = local write "单选_DSP_7"(w25) -> ()
        n310 = local write "单选_DSP_8"(w25) -> ()
        n311 = local write "单选_DSP_9"(w25) -> ()
        n312 = local write "单选_DSP_10"(w25) -> ()
        n313 = local write "单选_DSP_11"(w25) -> ()
        n314 = local write "单选_DSP_12"(w25) -> ()
        n315 = local write "单选_DSP_13"(w25) -> ()
        n316 = local write "单选_DSP_14"(w25) -> ()
        n317 = local write "单选_DSP_15"(w25) -> ()
        n318 = local write "单选_DSP_16"(w25) -> ()
      }
      event "btn_反选": Value Change {
        n319 = event-data() -> ()  [unwired: 1 in, 5 out]
        n320 = local read "单选_DSP_1"() -> (w57:bool)
        n321 = local read "单选_DSP_2"() -> (w55:bool)
        n322 = local read "单选_DSP_3"() -> (w54:bool)
        n323 = local read "单选_DSP_4"() -> (w53:bool)
        n324 = local read "单选_DSP_5"() -> (w52:bool)
        n325 = local read "单选_DSP_6"() -> (w51:bool)
        n326 = local read "单选_DSP_7"() -> (w50:bool)
        n327 = local read "单选_DSP_8"() -> (w49:bool)
        n328 = local read "单选_DSP_9"() -> (w48:bool)
        n329 = local read "单选_DSP_10"() -> (w47:bool)
        n330 = local read "单选_DSP_11"() -> (w46:bool)
        n331 = local read "单选_DSP_12"() -> (w45:bool)
        n332 = local read "单选_DSP_13"() -> (w44:bool)
        n333 = local read "单选_DSP_14"() -> (w43:bool)
        n334 = local read "单选_DSP_15"() -> (w42:bool)
        n335 = local read "单选_DSP_16"() -> (w41:bool)
        n336 = Not(x=w57) -> (.not. x?=w56:bool)
        n337 = Not(x=w55) -> (.not. x?=w26:bool)
        n338 = Not(x=w54) -> (.not. x?=w27:bool)
        n339 = Not(x=w53) -> (.not. x?=w28:bool)
        n340 = Not(x=w52) -> (.not. x?=w29:bool)
        n341 = Not(x=w51) -> (.not. x?=w30:bool)
        n342 = Not(x=w50) -> (.not. x?=w31:bool)
        n343 = Not(x=w49) -> (.not. x?=w32:bool)
        n344 = Not(x=w48) -> (.not. x?=w33:bool)
        n345 = Not(x=w47) -> (.not. x?=w34:bool)
        n346 = Not(x=w46) -> (.not. x?=w35:bool)
        n347 = Not(x=w45) -> (.not. x?=w36:bool)
        n348 = Not(x=w44) -> (.not. x?=w37:bool)
        n349 = Not(x=w43) -> (.not. x?=w38:bool)
        n350 = Not(x=w42) -> (.not. x?=w39:bool)
        n351 = Not(x=w41) -> (.not. x?=w40:bool)
        n352 = local write "单选_DSP_1"(w56) -> ()
        n353 = local write "单选_DSP_2"(w26) -> ()
        n354 = local write "单选_DSP_3"(w27) -> ()
        n355 = local write "单选_DSP_4"(w28) -> ()
        n356 = local write "单选_DSP_5"(w29) -> ()
        n357 = local write "单选_DSP_6"(w30) -> ()
        n358 = local write "单选_DSP_7"(w31) -> ()
        n359 = local write "单选_DSP_8"(w32) -> ()
        n360 = local write "单选_DSP_9"(w33) -> ()
        n361 = local write "单选_DSP_10"(w34) -> ()
        n362 = local write "单选_DSP_11"(w35) -> ()
        n363 = local write "单选_DSP_12"(w36) -> ()
        n364 = local write "单选_DSP_13"(w37) -> ()
        n365 = local write "单选_DSP_14"(w38) -> ()
        n366 = local write "单选_DSP_15"(w39) -> ()
        n367 = local write "单选_DSP_16"(w40) -> ()
      }
    }
    n368 = local write "退出？"(w1) -> ()
  }
  n369 = stacked-sequence {
    frame #0 {
      w62 = cluster{u32, u32}[] [{9868950, 9868950}]
      n370 = local write "开始时间"(0.0 ("开始时间")) -> ()
      n371 = property on="light_1" class="Bool (严格)"("Colors [4]"=w62) -> ()  [unwired: 2 in, 2 out]
      n372 = property on="light_2" class="Bool (严格)"("Colors [4]"=w62) -> ()  [unwired: 2 in, 2 out]
      n373 = property on="light_3" class="Bool (严格)"("Colors [4]"=w62) -> ()  [unwired: 2 in, 2 out]
      n374 = property on="light_4" class="Bool (严格)"("Colors [4]"=w62) -> ()  [unwired: 2 in, 2 out]
      n375 = property on="light_5" class="Bool (严格)"("Colors [4]"=w62) -> ()  [unwired: 2 in, 2 out]
      n376 = property on="light_6" class="Bool (严格)"("Colors [4]"=w62) -> ()  [unwired: 2 in, 2 out]
      n377 = property on="light_7" class="Bool (严格)"("Colors [4]"=w62) -> ()  [unwired: 2 in, 2 out]
      n378 = property on="light_8" class="Bool (严格)"("Colors [4]"=w62) -> ()  [unwired: 2 in, 2 out]
      n379 = property on="light_9" class="Bool (严格)"("Colors [4]"=w62) -> ()  [unwired: 2 in, 2 out]
      n380 = property on="light_10" class="Bool (严格)"("Colors [4]"=w62) -> ()  [unwired: 2 in, 2 out]
      n381 = property on="light_11" class="Bool (严格)"("Colors [4]"=w62) -> ()  [unwired: 2 in, 2 out]
      n382 = property on="light_12" class="Bool (严格)"("Colors [4]"=w62) -> ()  [unwired: 2 in, 2 out]
      n383 = property on="light_13" class="Bool (严格)"("Colors [4]"=w62) -> ()  [unwired: 2 in, 2 out]
      n384 = property on="light_14" class="Bool (严格)"("Colors [4]"=w62) -> ()  [unwired: 2 in, 2 out]
      n385 = property on="light_15" class="Bool (严格)"("Colors [4]"=w62) -> ()  [unwired: 2 in, 2 out]
      n386 = property on="light_16" class="Bool (严格)"("Colors [4]"=w62) -> ()  [unwired: 2 in, 2 out]
      n387 = Initialize Array(FALSE, 5 ("维数大小"), 16 ("维数大小")) -> (w58:bool[][])
      n388 = local write "合格？"(w58) -> ()
    }
  }
  n389 = while {
    stop <- w65 stop-if-true
    w68 = "DSPStart" ("名称（未命名）")
    n390 = Wait Until Next ms Multiple(millisecond multiple=u32 200 ("毫秒倍数")) -> ()  [unwired: 1 out]
    n391 = Obtain Notifier(name (unnamed)=w68, notification data type=w68) -> (notifier out=w74:refnum<notifier>, error out=w73:errorcluster)  [unwired: 2 in, 1 out]
    n392 = Wait on Notification(notifier=w74, timeout in ms (-1)=10 ("超时毫秒(-1)"), error in (no error)=w73) -> (notifier out=w72:refnum<notifier>, notification=w70:string, error out=w71:errorcluster)  [unwired: 1 in, 1 out]
    n393 = Equal?(x=w70, y="DSP" ("通知")) -> (x = y?=w66:bool)
    n394 = Release Notifier(notifier=w72, error in (no error)=w71) -> ()  [unwired: 1 in, 3 out]
    n395 = case shown="真" w66 {
      frame False {
      }
      frame True {
        n396 = stacked-sequence {
          frame #0 {
            # "模拟量输入"
            n397 = for {
              N: 8 -> [_]
              i -> [w76]
              n398 = case shown="0, 默认" w76 {
                frame 1 {
                  n399 = for {
                    N: 5 -> [_]
                    i -> [w83]
                    n400 = case shown="4" w83 {
                      tunnel: [w85 w87 w89 w91 w93] -> w82
                      tunnel: [w84 w86 w88 w90 w92] -> w81
                      frame 0, Default {
                        n401 = local read "DSP_3_1"() -> (w85:sgl)
                        n402 = local read "DSP_4_1"() -> (w84:sgl)
                      }
                      frame 1 {
                        n403 = local read "DSP_3_2"() -> (w87:sgl)
                        n404 = local read "DSP_4_2"() -> (w86:sgl)
                      }
                      frame 2 {
                        n405 = local read "DSP_3_3"() -> (w89:sgl)
                        n406 = local read "DSP_4_3"() -> (w88:sgl)
                      }
                      frame 3 {
                        n407 = local read "DSP_3_4"() -> (w91:sgl)
                        n408 = local read "DSP_4_4"() -> (w90:sgl)
                      }
                      frame 4 {
                        n409 = local read "DSP_3_5"() -> (w93:sgl)
                        n410 = local read "DSP_4_5"() -> (w92:sgl)
                      }
                    }
                    n411 = local read "单选_DSP_3"() -> (w78:bool)
                    n412 = local read "单选_DSP_4"() -> (w79:bool)
                    n413 = call "两路模拟量输入.vi"("第2路值"=w81, "选择第2路？"=w79, "第1路值"=w82, "选择第1路？"=w78) -> ("选择？"=w80:bool)  [unwired: 7 in]
                    n414 = case shown="真" w80 {
                      frame False {
                      }
                      frame True {
                        n415 = call "时间延迟3"() -> ()  [unwired: 11 in, 1 out]
                      }
                    }
                  }
                }
                frame 2 {
                  n416 = for {
                    N: 5 -> [_]
                    i -> [w100]
                    n417 = case shown="4" w100 {
                      tunnel: [w102 w104 w106 w108 w110] -> w99
                      tunnel: [w101 w103 w105 w107 w109] -> w98
                      frame 0, Default {
                        n418 = local read "DSP_5_1"() -> (w102:sgl)
                        n419 = local read "DSP_6_1"() -> (w101:sgl)
                      }
                      frame 1 {
                        n420 = local read "DSP_5_2"() -> (w104:sgl)
                        n421 = local read "DSP_6_2"() -> (w103:sgl)
                      }
                      frame 2 {
                        n422 = local read "DSP_5_3"() -> (w106:sgl)
                        n423 = local read "DSP_6_3"() -> (w105:sgl)
                      }
                      frame 3 {
                        n424 = local read "DSP_5_4"() -> (w108:sgl)
                        n425 = local read "DSP_6_4"() -> (w107:sgl)
                      }
                      frame 4 {
                        n426 = local read "DSP_5_5"() -> (w110:sgl)
                        n427 = local read "DSP_6_5"() -> (w109:sgl)
                      }
                    }
                    n428 = local read "单选_DSP_5"() -> (w96:bool)
                    n429 = local read "单选_DSP_6"() -> (w95:bool)
                    n430 = call "两路模拟量输入.vi"("第2路值"=w98, "选择第2路？"=w95, "第1路值"=w99, "选择第1路？"=w96) -> ("选择？"=w97:bool)  [unwired: 7 in]
                    n431 = case shown="真" w97 {
                      frame False {
                      }
                      frame True {
                        n432 = call "时间延迟4"() -> ()  [unwired: 11 in, 1 out]
                      }
                    }
                  }
                }
                frame 3 {
                  n433 = for {
                    N: 5 -> [_]
                    i -> [w117]
                    n434 = case shown="4" w117 {
                      tunnel: [w119 w121 w123 w125 w127] -> w116
                      tunnel: [w118 w120 w122 w124 w126] -> w115
                      frame 0, Default {
                        n435 = local read "DSP_7_1"() -> (w119:sgl)
                        n436 = local read "DSP_8_1"() -> (w118:sgl)
                      }
                      frame 1 {
                        n437 = local read "DSP_7_2"() -> (w121:sgl)
                        n438 = local read "DSP_8_2"() -> (w120:sgl)
                      }
                      frame 2 {
                        n439 = local read "DSP_7_3"() -> (w123:sgl)
                        n440 = local read "DSP_8_3"() -> (w122:sgl)
                      }
                      frame 3 {
                        n441 = local read "DSP_7_4"() -> (w125:sgl)
                        n442 = local read "DSP_8_4"() -> (w124:sgl)
                      }
                      frame 4 {
                        n443 = local read "DSP_7_5"() -> (w127:sgl)
                        n444 = local read "DSP_8_5"() -> (w126:sgl)
                      }
                    }
                    n445 = local read "单选_DSP_7"() -> (w113:bool)
                    n446 = local read "单选_DSP_8"() -> (w112:bool)
                    n447 = call "两路模拟量输入.vi"("第2路值"=w115, "选择第2路？"=w112, "第1路值"=w116, "选择第1路？"=w113) -> ("选择？"=w114:bool)  [unwired: 7 in]
                    n448 = case shown="真" w114 {
                      frame False {
                      }
                      frame True {
                        n449 = call "时间延迟5"() -> ()  [unwired: 11 in, 1 out]
                      }
                    }
                  }
                }
                frame 4 {
                  n450 = for {
                    N: 5 -> [_]
                    i -> [w134]
                    n451 = case shown="4" w134 {
                      tunnel: [w136 w138 w140 w142 w144] -> w133
                      tunnel: [w135 w137 w139 w141 w143] -> w132
                      frame 0, Default {
                        n452 = local read "DSP_9_1"() -> (w136:sgl)
                        n453 = local read "DSP_10_1"() -> (w135:sgl)
                      }
                      frame 1 {
                        n454 = local read "DSP_9_2"() -> (w138:sgl)
                        n455 = local read "DSP_10_2"() -> (w137:sgl)
                      }
                      frame 2 {
                        n456 = local read "DSP_9_3"() -> (w140:sgl)
                        n457 = local read "DSP_10_3"() -> (w139:sgl)
                      }
                      frame 3 {
                        n458 = local read "DSP_9_4"() -> (w142:sgl)
                        n459 = local read "DSP_10_4"() -> (w141:sgl)
                      }
                      frame 4 {
                        n460 = local read "DSP_9_5"() -> (w144:sgl)
                        n461 = local read "DSP_10_5"() -> (w143:sgl)
                      }
                    }
                    n462 = local read "单选_DSP_10"() -> (w129:bool)
                    n463 = local read "单选_DSP_9"() -> (w130:bool)
                    n464 = call "两路模拟量输入.vi"("第2路值"=w132, "选择第2路？"=w129, "第1路值"=w133, "选择第1路？"=w130) -> ("选择？"=w131:bool)  [unwired: 7 in]
                    n465 = case shown="真" w131 {
                      frame False {
                      }
                      frame True {
                        n466 = call "时间延迟6"() -> ()  [unwired: 11 in, 1 out]
                      }
                    }
                  }
                }
                frame 5 {
                  n467 = for {
                    N: 5 -> [_]
                    i -> [w151]
                    n468 = case shown="4" w151 {
                      tunnel: [w153 w155 w157 w159 w161] -> w150
                      tunnel: [w152 w154 w156 w158 w160] -> w149
                      frame 0, Default {
                        n469 = local read "DSP_11_1"() -> (w153:sgl)
                        n470 = local read "DSP_12_1"() -> (w152:sgl)
                      }
                      frame 1 {
                        n471 = local read "DSP_11_2"() -> (w155:sgl)
                        n472 = local read "DSP_12_2"() -> (w154:sgl)
                      }
                      frame 2 {
                        n473 = local read "DSP_11_3"() -> (w157:sgl)
                        n474 = local read "DSP_12_3"() -> (w156:sgl)
                      }
                      frame 3 {
                        n475 = local read "DSP_11_4"() -> (w159:sgl)
                        n476 = local read "DSP_12_4"() -> (w158:sgl)
                      }
                      frame 4 {
                        n477 = local read "DSP_11_5"() -> (w161:sgl)
                        n478 = local read "DSP_12_5"() -> (w160:sgl)
                      }
                    }
                    n479 = local read "单选_DSP_11"() -> (w147:bool)
                    n480 = local read "单选_DSP_12"() -> (w146:bool)
                    n481 = call "两路模拟量输入.vi"("第2路值"=w149, "选择第2路？"=w146, "第1路值"=w150, "选择第1路？"=w147) -> ("选择？"=w148:bool)  [unwired: 7 in]
                    n482 = case shown="真" w148 {
                      frame False {
                      }
                      frame True {
                        n483 = call "时间延迟7"() -> ()  [unwired: 11 in, 1 out]
                      }
                    }
                  }
                }
                frame 6 {
                  n484 = for {
                    N: 5 -> [_]
                    i -> [w168]
                    n485 = case shown="4" w168 {
                      tunnel: [w170 w172 w174 w176 w178] -> w167
                      tunnel: [w169 w171 w173 w175 w177] -> w166
                      frame 0, Default {
                        n486 = local read "DSP_13_1"() -> (w170:sgl)
                        n487 = local read "DSP_6_14"() -> (w169:sgl)
                      }
                      frame 1 {
                        n488 = local read "DSP_13_2"() -> (w172:sgl)
                        n489 = local read "DSP_14_2"() -> (w171:sgl)
                      }
                      frame 2 {
                        n490 = local read "DSP_13_3"() -> (w174:sgl)
                        n491 = local read "DSP_14_3"() -> (w173:sgl)
                      }
                      frame 3 {
                        n492 = local read "DSP_13_4"() -> (w176:sgl)
                        n493 = local read "DSP_14_4"() -> (w175:sgl)
                      }
                      frame 4 {
                        n494 = local read "DSP_13_5"() -> (w178:sgl)
                        n495 = local read "DSP_14_5"() -> (w177:sgl)
                      }
                    }
                    n496 = local read "单选_DSP_13"() -> (w163:bool)
                    n497 = local read "单选_DSP_14"() -> (w164:bool)
                    n498 = call "两路模拟量输入.vi"("第2路值"=w166, "选择第2路？"=w164, "第1路值"=w167, "选择第1路？"=w163) -> ("选择？"=w165:bool)  [unwired: 7 in]
                    n499 = case shown="真" w165 {
                      frame False {
                      }
                      frame True {
                        n500 = call "时间延迟8"() -> ()  [unwired: 11 in, 1 out]
                      }
                    }
                  }
                }
                frame 7 {
                  n501 = for {
                    N: 5 -> [_]
                    i -> [w185]
                    n502 = case shown="4" w185 {
                      tunnel: [w187 w189 w191 w193 w195] -> w184
                      tunnel: [w186 w188 w190 w192 w194] -> w183
                      frame 0, Default {
                        n503 = local read "DSP_15_1"() -> (w187:sgl)
                        n504 = local read "DSP_16_1"() -> (w186:sgl)
                      }
                      frame 1 {
                        n505 = local read "DSP_15_2"() -> (w189:sgl)
                        n506 = local read "DSP_16_2"() -> (w188:sgl)
                      }
                      frame 2 {
                        n507 = local read "DSP_15_3"() -> (w191:sgl)
                        n508 = local read "DSP_16_3"() -> (w190:sgl)
                      }
                      frame 3 {
                        n509 = local read "DSP_15_4"() -> (w193:sgl)
                        n510 = local read "DSP_16_4"() -> (w192:sgl)
                      }
                      frame 4 {
                        n511 = local read "DSP_15_5"() -> (w195:sgl)
                        n512 = local read "DSP_16_5"() -> (w194:sgl)
                      }
                    }
                    n513 = local read "单选_DSP_15"() -> (w181:bool)
                    n514 = local read "单选_DSP_16"() -> (w180:bool)
                    n515 = call "两路模拟量输入.vi"("第2路值"=w183, "选择第2路？"=w180, "第1路值"=w184, "选择第1路？"=w181) -> ("选择？"=w182:bool)  [unwired: 7 in]
                    n516 = case shown="真" w182 {
                      frame False {
                      }
                      frame True {
                        n517 = call "时间延迟2"() -> ()  [unwired: 11 in, 1 out]
                      }
                    }
                  }
                }
                frame 0, Default {
                  n518 = for {
                    N: 5 -> [_]
                    i -> [w202]
                    n519 = case shown="4" w202 {
                      tunnel: [w204 w206 w208 w210 w212] -> w201
                      tunnel: [w203 w205 w207 w209 w211] -> w200
                      frame 0, Default {
                        n520 = local read "DSP_1_1"() -> (w204:sgl)
                        n521 = local read "DSP_2_1"() -> (w203:sgl)
                      }
                      frame 1 {
                        n522 = local read "DSP_1_2"() -> (w206:sgl)
                        n523 = local read "DSP_2_2"() -> (w205:sgl)
                      }
                      frame 2 {
                        n524 = local read "DSP_1_3"() -> (w208:sgl)
                        n525 = local read "DSP_2_3"() -> (w207:sgl)
                      }
                      frame 3 {
                        n526 = local read "DSP_1_4"() -> (w210:sgl)
                        n527 = local read "DSP_2_4"() -> (w209:sgl)
                      }
                      frame 4 {
                        n528 = local read "DSP_1_5"() -> (w212:sgl)
                        n529 = local read "DSP_2_5"() -> (w211:sgl)
                      }
                    }
                    n530 = local read "单选_DSP_1"() -> (w198:bool)
                    n531 = local read "单选_DSP_2"() -> (w197:bool)
                    n532 = call "两路模拟量输入.vi"("第2路值"=w200, "选择第2路？"=w197, "第1路值"=w201, "选择第1路？"=w198) -> ("选择？"=w199:bool)  [unwired: 7 in]
                    n533 = case shown="真" w199 {
                      frame False {
                      }
                      frame True {
                        n534 = call "时间延迟"() -> ()  [unwired: 11 in, 1 out]
                      }
                    }
                  }
                }
              }
            }
          }
          frame #1 {
            w214 = "DSPCheck" ("名称（未命名）")
            n535 = Obtain Notifier(name (unnamed)=w214, notification data type=w214) -> (notifier out=w213:refnum<notifier>)  [unwired: 2 in, 2 out]
            n536 = Send Notification(notification="check" ("通知"), notifier=w213) -> ()  [unwired: 1 in, 2 out]
          }
        }
      }
    }
    n537 = local read "退出？"() -> (w65:bool)
  }
  n538 = while {
    stop <- w226 stop-if-true
    w223 = "DSPCheck" ("名称（未命名）")
    # "校验"
    n539 = Wait Until Next ms Multiple(millisecond multiple=u32 200 ("毫秒倍数")) -> ()  [unwired: 1 out]
    n540 = Obtain Notifier(name (unnamed)=w223, notification data type=w223) -> (notifier out=w218:refnum<notifier>, error out=w219:errorcluster)  [unwired: 2 in, 1 out]
    n541 = Wait on Notification(notifier=w218, timeout in ms (-1)=10 ("超时毫秒(-1)"), error in (no error)=w219) -> (notifier out=w220:refnum<notifier>, notification=w222:string, error out=w221:errorcluster)  [unwired: 1 in, 1 out]
    n542 = Equal?(x=w222, y="check" ("通知")) -> (x = y?=w217:bool)
    n543 = Release Notifier(notifier=w220, error in (no error)=w221) -> ()  [unwired: 1 in, 3 out]
    n544 = case shown="真" w217 {
      frame False {
      }
      frame True {
      }
    }
    n545 = local read "退出？"() -> (w226:bool)
  }
